vi "Get Phys Instrs.vi"(11 "MSS in":refnum<class "Measure and Stimulus Subsystems.lvclass">) -> (2 "Phys Instr":T1(c390), 3 "MSS out":refnum<class "Measure and Stimulus Subsystems.lvclass">)   [LabVIEW 2023, in "HAL GOOP4.lvlib" / "Measure and Stimulus Subsystems.lvclass"]
uses:
  Measure and Stimulus Subsystems.lvclass
  Instrument/Instrument.lvclass
  Measure and Stimulus Subsystems.lvclass/Measure and Stimulus Subsystems.ctl
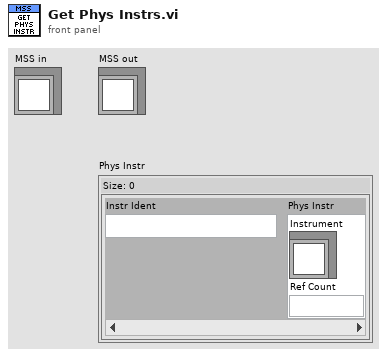
[diagram p1: front panel]
types:
  T1 = map{string, cluster{"Instrument":refnum<class "Instrument.lvclass">, "Ref Count":u8}}
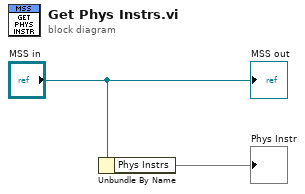
[diagram p0: block diagram]
diagram:
  n1 = Unbundle By Name("MSS in") -> ("Phys Instrs"=→"Phys Instr":T1)
  "MSS out" <- "MSS in"
